vi "Get Report Settings.vi"(0 "report in":refnum<class "NI_report.lvclass">, 11 "error in (no error)":errorcluster) -> (4 "report out":refnum<class "NI_report.lvclass">, 6 "text options":T1, 10 "font settings":T2, 14 "text color":u32(colorbox), 15 "error out":errorcluster)   [LabVIEW 2015, in "NI_report.lvclass"]
doc: "Retrieves information about the current font and text settings of a given report."
uses:
  <vilib>/Utility/NIReport.llb/NI_report.lvclass
panel:
  out "color - RGB":cluster{"red":u8, "green":u8, "blue":u8}
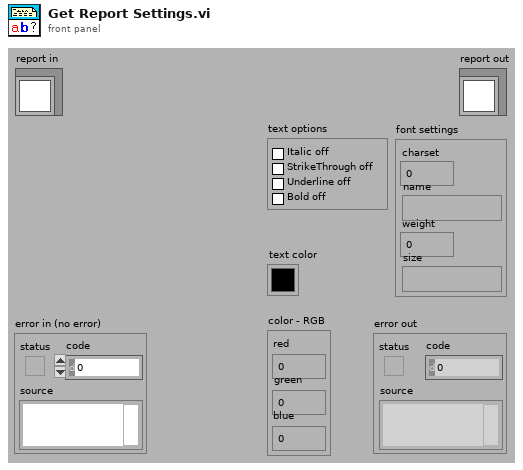
[diagram p1: front panel]
types:
  T1 = cluster{"Italic":bool, "StrikeThrough":bool, "Underline":bool, "Bold":bool}
  T2 = cluster{"charset":i16, "name":string, "weight":i16, "size":string}
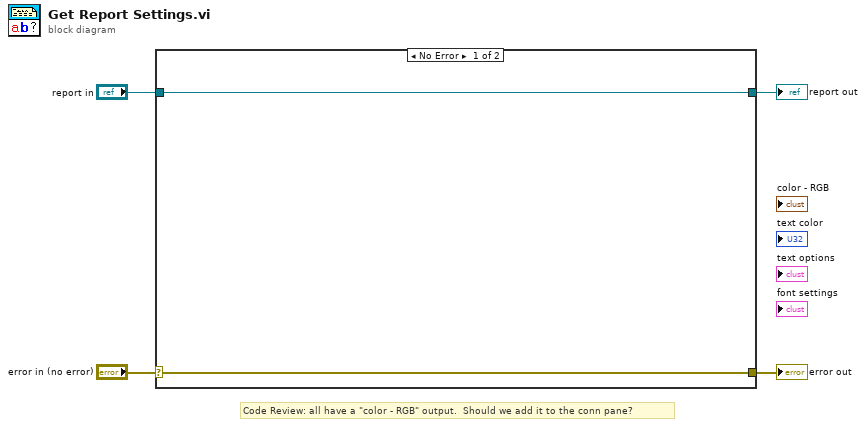
[diagram p0: block diagram]
diagram:
  # "Code Review: all have a \"color - RGB\" output.  Should we add it to the conn pane?"
  n1 = case shown="No Error" "error in (no error)" {
    selector: "error in (no error)" -> [w5 w8]
    tunnel: [w5 w8] -> w3
    tunnel: [w6 w7] -> w1
    tunnel: "report in" -> [w6 w7]
    frame No Error {
    }
    frame Error {
    }
  }
  "error out" <- w3
  "report out" <- w1
